vi "image decryption.vi"() -> ()   [LabVIEW 2022 SP3]
uses:
  <vilib>/picture/picture.llb/Draw True-Color Pixmap.vi
  index values of B.vi
  index Values of R.vi
  index Values of G.vi
  Row size.vi
  Column size.vi
panel:
  out "DATA IMAGE EXTRACTED":picture
  out "Data image B values":u8[][](array[numeric])
  out "Data image G values":u8[][](array[numeric])
  out "Data image R values":u8[][](array[numeric])
  out "COVER IMAGE":picture
  in  "Encoding Cover image Path":path
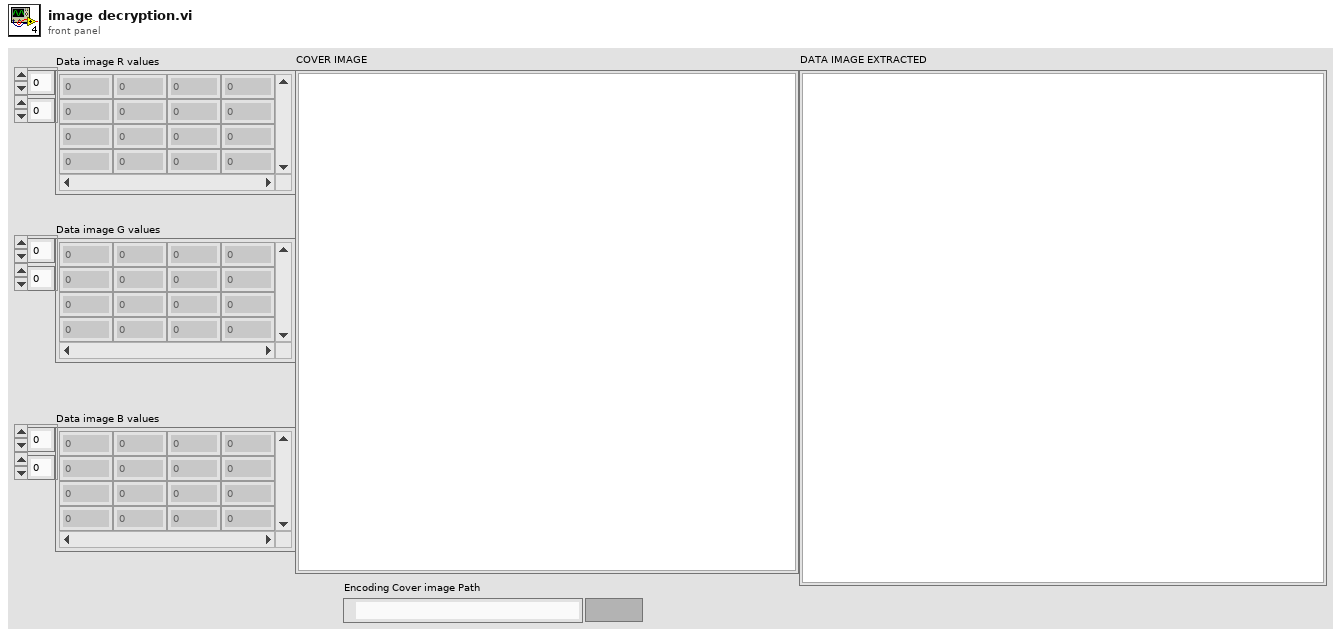
[diagram p1: front panel]
types:
  T1 = typedef "imagedata.ctl" = cluster{"image type":i32, "image depth":i32, "image":u8[], "mask":u8[], "colors":u32[], "Rectangle":cluster{"left":i16, "top":i16, "right":i16, "bottom":i16}}
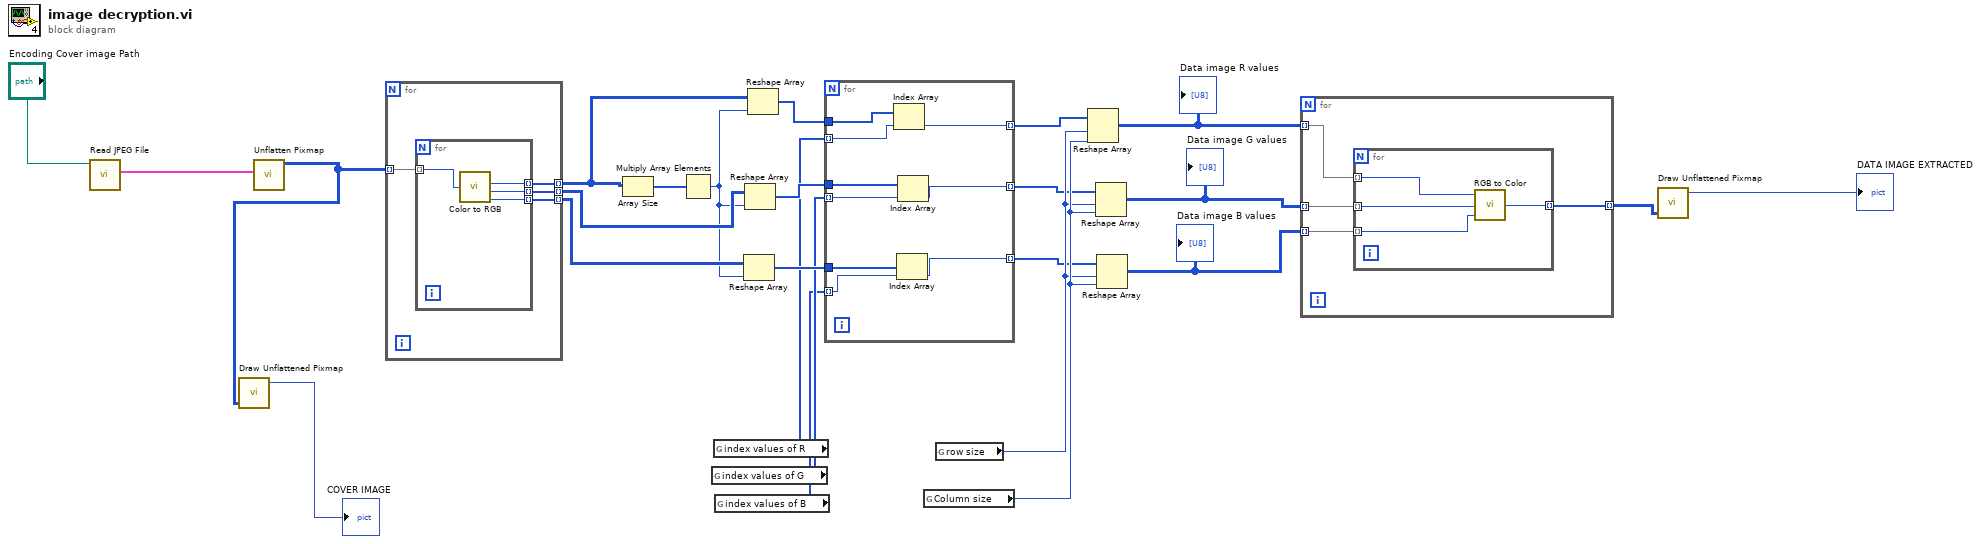
[diagram p0: block diagram]
diagram:
  n1 = call <vilib>:"Read JPEG File.vi"("path to JPEG file"="Encoding Cover image Path") -> ("image data"=w24:T1)  [unwired: 8 in, 2 out]
  n2 = call <vilib>:"Unflatten Pixmap.vi"("image data"=w24) -> ("24-bit pixmap"=w2:u32[][])  [unwired: 4 in, 6 out]
  n3 = call-poly <vilib>:"Draw Unflattened Pixmap.vi"("data (RGB format)"=w2) -> ("new picture"=→"COVER IMAGE":picture)  [unwired: 8 in]
  n4 = for {
    tunnel: w2 -> [w29] mode=indexing
    tunnel: [w28] -> w21 mode=indexing
    tunnel: [w27] -> w23 mode=indexing
    tunnel: [w26] -> w22 mode=indexing
    n5 = for {
      tunnel: w29 -> [w33] mode=indexing
      tunnel: [w32] -> w28 mode=indexing
      tunnel: [w31] -> w27 mode=indexing
      tunnel: [w30] -> w26 mode=indexing
      n6 = call <vilib>:"Color to RGB.vi"("Color"=w33) -> ("R"=w32:u8, "G"=w31:u8, "B"=w30:u8)  [unwired: 1 out]
    }
  }
  n7 = Array Size(array=w21) -> (size(s)=w20:i32[])
  n8 = Multiply Array Elements(1:w20) -> (0:w19:i32)
  n9 = global read "index Values of G.vi" "index values of G"() -> (w14:i32[])
  n10 = global read "index Values of R.vi" "index values of R"() -> (w15:i32[])
  n11 = global read "index values of B.vi" "index values of B"() -> (w13:i32[])
  n12 = Reshape Array(w22, w19) -> (w16:u8[])
  n13 = Reshape Array(w23, w19) -> (w17:u8[])
  n14 = Reshape Array "Reshape Array"(w21, w19) -> (w18:u8[])
  n15 = for {
    tunnel: w18 -> [w42]
    tunnel: w17 -> [w41]
    tunnel: w16 -> [w40]
    tunnel: w15 -> [w39] mode=indexing
    tunnel: w14 -> [w38] mode=indexing
    tunnel: w13 -> [w37] mode=indexing
    tunnel: [w36] -> w10 mode=indexing
    tunnel: [w35] -> w9 mode=indexing
    tunnel: [w34] -> w8 mode=indexing
    n16 = Index Array(array=w42, index=w39) -> (element=w35:u8)
    n17 = Index Array(array=w40, index=w37) -> (element=w34:u8)
    n18 = Index Array "Index Array"(array=w41, index=w38) -> (element=w36:u8)
  }
  n19 = global read "Column size.vi" "Column size"() -> (w12:i32)
  n20 = global read "Row size.vi" "row size"() -> (w11:i32)
  n21 = Reshape Array(w9, w11, w12) -> (w7:u8[][])
  "Data image R values" <- w7
  n22 = Reshape Array "Reshape Array"(w10, w11, w12) -> (w6:u8[][])
  "Data image G values" <- w6
  n23 = Reshape Array(w8, w11, w12) -> (w5:u8[][])
  "Data image B values" <- w5
  n24 = for {
    tunnel: w7 -> [w46] mode=indexing
    tunnel: w6 -> [w45] mode=indexing
    tunnel: w5 -> [w44] mode=indexing
    tunnel: [w43] -> w4 mode=indexing
    n25 = for {
      tunnel: w46 -> [w50] mode=indexing
      tunnel: w45 -> [w49] mode=indexing
      tunnel: w44 -> [w48] mode=indexing
      tunnel: [w47] -> w43 mode=indexing
      n26 = call <vilib>:"RGB to Color.vi"("B"=w48, "G"=w49, "R"=w50) -> ("Color"=w47:u32)
    }
  }
  n27 = call-poly <vilib>:"Draw Unflattened Pixmap.vi"("data (RGB format)"=w4) -> ("new picture"=→"DATA IMAGE EXTRACTED":picture)  [unwired: 8 in]
